vi "Main Tclk.vi"() -> ()   [LabVIEW 2018] (continued)
                      tunnel: [w9192] -> w9169 mode=indexing
                      tunnel: [w9191] -> w9167 mode=indexing
                      tunnel: [w9190] -> w9166 mode=indexing
                      i -> [w9198]
                      n3011 = for {
                        tunnel: w9204 -> [w9220] mode=indexing
                        tunnel: w9203 -> [w9219] mode=indexing
                        tunnel: w9202 -> [w9218]
                        tunnel: w9201 -> [w9217] mode=indexing
                        tunnel: w9200 -> [w9216]
                        tunnel: [w9215] -> w9199 mode=indexing
                        tunnel: w9198 -> [w9214]
                        tunnel: [w9212] -> w9197 mode=indexing
                        tunnel: [w9211] -> w9196 mode=indexing
                        tunnel: [w9210] -> w9195 mode=indexing
                        tunnel: [w9209] -> w9194 mode=indexing
                        tunnel: w9193 -> [w9208]
                        tunnel: [w9207] -> w9192 mode=indexing
                        tunnel: [w9206] -> w9191 mode=indexing
                        tunnel: [w9205] -> w9190 mode=indexing
                        i -> [w9213]
                        n3012 = stacked-sequence {
                          seq-local: [w9223 _ _] -> [_ w9261 _]
                          seq-local: [w9221 _ _] -> [_ w9252 _]
                          tunnel: w9220 -> [w9228 w9253 w9308]
                          tunnel: w9219 -> [w9227 w9266 w9307]
                          tunnel: w9218 -> [w9225 w9249 _]
                          tunnel: w9217 -> [w9222 _ _]
                          tunnel: w9216 -> [w9224 w9250 _]
                          tunnel: [_ w9262 _] -> w9215
                          tunnel: w9214 -> [_ w9260 _]
                          tunnel: w9213 -> [_ w9259 _]
                          tunnel: [w9221 _ _] -> w9212
                          tunnel: [_ w9258 _] -> w9211
                          tunnel: [_ w9257 _] -> w9210
                          tunnel: [_ w9256 _] -> w9209
                          tunnel: w9208 -> [_ w9255 _]
                          tunnel: [_ w9254 _] -> w9207
                          tunnel: [_ w9251 _] -> w9206
                          tunnel: [_ _ w9306] -> w9205
                          frame #0 {
                            n3013 = Subtract(x=w9224, y=w9222) -> (x-y=w9226:u8)
                            n3014 = Less?(x=w9225, y=w9226) -> (x < y?=w9229:bool)
                            n3015 = case shown="True" w9229 {
                              tunnel: w9228 -> [w9231 w9236]
                              tunnel: w9225 -> [_ w9235]
                              tunnel: w9227 -> [_ w9237]
                              tunnel: [w9231 w9234] -> w9223
                              tunnel: w9222 -> [w9230 w9233]
                              tunnel: [w9230 w9232] -> w9221
                              frame False {
                              }
                              frame True {
                                n3016 = Index Array(array=w9236, index=w9235) -> (element=w9239:sgl)
                                n3017 = call "1D Parabolic Max.vi"("Y"=w9237, "Xt"=w9239, "X"=w9236) -> ("Y(Xt) < Ymin"=w9238:bool)  [unwired: 1 in, 7 out]
                                n3018 = case shown="False" w9238 {
                                tunnel: w9235 -> [_ w9245]
                                tunnel: w9236 -> [w9241 w9246]
                                tunnel: w9233 -> [w9240 w9243]
                                tunnel: [w9241 w9244] -> w9234
                                tunnel: [w9240 w9242] -> w9232
                                frame False {
                                }
                                frame True {
                                n3019 = Delete From Array(array=w9246, length=1, index=w9245) -> (array with subset deleted=w9244:sgl[])  [unwired: 1 out]
                                n3020 = Increment(x=w9243) -> (x+1=w9242:u8)
                                }
                                }
                              }
                            }
                          }
                          frame #1 {
                            n3021 = Subtract(x=w9250, y=w9252) -> (x-y=w9265:u8)
                            n3022 = call "1D Parabolic Max.vi"("Y"=w9266, "X"=w9253) -> ("Found max"=w9256:bool, "Ymax"=w9263:dbl, "Xmax"=w9267:dbl, "Finer Best Polynomial Fit"=w9269:dbl[], "Finer X"=w9264:dbl[])  [unwired: 2 in, 3 out]
                            n3023 = Greater Or Equal?(x=w9249, y=w9265) -> (x >= y?=w9268:bool)
                            n3024 = Subtract(x=w9250, y=w9249) -> (x-y=w9248:u8)
                            n3025 = Compound Arithmetic op=OR(w9256, w9268, w9255) -> (w9254:bool)
                            n3026 = case shown="True" w9254 {
                              tunnel: w9267 -> [_ w9287]
                              tunnel: w9266 -> [w9271 w9299]
                              tunnel: w9261 -> [w9279 _]
                              tunnel: w9269 -> [_ w9298]
                              tunnel: w9264 -> [_ w9297]
                              tunnel: w9263 -> [_ w9288]
                              tunnel: w9248 -> [_ w9296]
                              tunnel: w9249 -> [_ w9294]
                              tunnel: [w9279 w9293] -> w9262
                              tunnel: w9260 -> [w9276 w9284]
                              tunnel: w9259 -> [w9277 w9283]
                              tunnel: [w9270 w9288] -> w9258
                              tunnel: [w9274 w9287] -> w9257
                              tunnel: w9253 -> [w9275 w9286]
                              tunnel: [w9278 w9285] -> w9251
                              frame False {
                                n3027 = Build Cluster Array(w9275, w9271) -> (w9280:cluster{"Center":sgl, "A Img Focus Index":sgl}[])
                                n3028 = Sort 1D Array(array=w9280) -> (sorted array=w9281:cluster{"Center":sgl, "A Img Focus Index":sgl}[])
                                n3029 = Bundle(w9281) -> (w9282:T73)  [unwired: 1 in]
                                n3030 = Build Array(w9282) -> (w9278:T74)
                                n3031 = local write "AAX Y tile"(w9276) -> ()
                                n3032 = local write "AAX X tile"(w9277) -> ()
                                n3033 = local write "Auto Aln X"(w9278) -> ()
                                n3034 = Index Array(array=w9275, index=0) -> (element=w9274:sgl)
                                n3035 = Index Array(array=w9271, index=0) -> (element=w9270:sgl)
                              }
                              frame True {
                                n3036 = local read "SEM Scan Parameters"() -> (w9291:T26)
                                n3037 = Initialize Array(w9287, w9296) -> (w9295:dbl[])
                                n3038 = Replace Array Subset(array=w9286, new element=w9295, index=w9294) -> (w9293:sgl[])
                                n3039 = Build Cluster Array(w9286, w9299) -> (w9304:cluster{"Center":sgl, "A Img Focus Index":sgl}[])
                                n3040 = Build Cluster Array(w9297, w9298) -> (w9301:cluster{dbl, dbl}[])
                                n3041 = local write "AAX Y tile"(w9284) -> ()
                                n3042 = local write "AAX X tile"(w9283) -> ()
                                n3043 = Unbundle By Name(w9291) -> ("X aln"=w9292:sgl[][])
                                n3044 = Sort 1D Array(array=w9304) -> (sorted array=w9303:cluster{"Center":sgl, "A Img Focus Index":sgl}[])
                                n3045 = Sort 1D Array(array=w9301) -> (sorted array=w9302:cluster{dbl, dbl}[])
                                n3046 = Replace Array Subset(array=w9292, new element=w9287, index (row)=w9284, index (col)=w9283) -> (w9290:sgl[][])
                                n3047 = Bundle(w9303) -> (w9305:T73)  [unwired: 1 in]
                                n3048 = Bundle(w9302) -> (w9300:cluster{cluster{dbl, dbl}[]})  [unwired: 1 in]
                                n3049 = Bundle By Name(cluster=w9291, "X aln"=w9290) -> (w9289:T26)
                                n3050 = local write "SEM Scan Parameters"(w9289) -> ()
                                n3051 = Build Array(w9305, w9300) -> (w9285:T75)
                                n3052 = local write "Auto Aln X"(w9285) -> ()
                              }
                            }
                          }
                          frame #2 {
                            n3053 = Array Size(array=w9307) -> (size(s)=w9310:i32)
                            n3054 = Greater Or Equal?(x=w9310, y=2) -> (x >= y?=w9311:bool)
                            n3055 = Array Subset(array=w9308, length=w9310) -> (w9309:sgl[])  [unwired: 1 in]
                            n3056 = case shown="True" w9311 {
                              tunnel: w9307 -> [_ w9323]
                              tunnel: w9309 -> [_ w9319]
                              tunnel: [_ w9313] -> w9306
                              frame False {
                              }
                              frame True {
                                n3057 = Array Max & Min(array=w9319) -> (max value=w9321:sgl, min value=w9320:sgl)  [unwired: 2 out]
                                n3058 = Array Max & Min(array=w9323) -> (max value=w9325:sgl, min value=w9326:sgl)  [unwired: 2 out]
                                n3059 = Subtract(x=w9321, y=w9320) -> (x-y=w9322:sgl)
                                n3060 = Subtract(x=w9325, y=w9326) -> (x-y=w9324:sgl)
                                n3061 = expression code="x*0.2"(w9322) -> (w9318:sgl)
                                n3062 = expression code="x*0.2"(w9324) -> (w9327:sgl)
                                n3063 = Add(x=w9321, y=w9318) -> (x+y=w9317:sgl)
                                n3064 = Subtract(x=w9320, y=w9318) -> (x-y=w9316:sgl)
                                n3065 = Add(x=w9325, y=w9327) -> (x+y=w9315:sgl)
                                n3066 = Subtract(x=w9326, y=w9327) -> (x-y=w9314:sgl)
                                n3067 = Bundle(w9317, w9316, w9315, w9314) -> (w9313:cluster{sgl, sgl, sgl, sgl})  [unwired: 1 in]
                                n3068 = property on="Auto Aln X" class="XYGraph (strict)"("XScale.Maximum"=w9317, "XScale.Minimum"=w9316, "YScale.Maximum"=w9315, "YScale.Minimum"=w9314) -> ()  [unwired: 2 in, 2 out]
                              }
                            }
                          }
                        }
                      }
                    }
                    n3069 = And Array Elements(Boolean array=w9169) -> (logical AND=w9168:bool)
                    n3070 = local write "AAX Success tiled"(w9171) -> ()
                    n3071 = local write "AAX Graph scales tiled"(w9166) -> ()
                    n3072 = local write "AlnX array tiled"(w9175) -> ()
                    n3073 = local write "AAX Graph tiled"(w9167) -> ()
                    n3074 = local write "Best Aln X FI tiled"(w9173) -> ()
                    n3075 = local write "Skip Steps tiled"(w9174) -> ()
                    n3076 = local write "Best Aln X (%) tiled"(w9172) -> ()
                    n3077 = case shown="True" w9168 {
                      frame False {
                      }
                      frame True {
                        w9187 = T44."Enabled" ("Disabled")
                        w9189 = sgl[][][] [] ("FI array tiled")
                        n3078 = local read "SEM Scan Parameters"() -> (w9186:T26)
                        n3079 = Unbundle By Name(w9186) -> ("Y tiles"=w9182:u8, "X tiles"=w9183:u8)
                        n3080 = local write "AA Count"(u8 0 ("AA Count")) -> ()
                        n3081 = local write "FI array tiled"(w9189) -> ()
                        n3082 = local write "AlnX array tiled"(w9189) -> ()
                        n3083 = local write "Aln Options"(enum16{"Defaut", "Aln X", "Aln Y"}."Aln Y" ("Aln Options")) -> ()
                        n3084 = property on="Auto Align" class="Bool (strict)"("DisabledEnum"=w9187) -> ()  [unwired: 2 in, 2 out]
                        n3085 = property on="AA Steps" class="DigNum (strict)"("DisabledEnum"=w9187) -> ()  [unwired: 2 in, 2 out]
                        n3086 = Initialize Array(u8 0 ("Skip Steps"), w9182, w9183) -> (w9184:u8[][])
                        n3087 = local write "Skip Steps tiled"(w9184) -> ()
                      }
                    }
                  }
                  frame True {
                  }
                }
              }
              frame #35 {
                n3088 = local read "AlnY array tiled"() -> (w9329:sgl[][][])
                n3089 = local read "FI array tiled"() -> (w9330:sgl[][][])
                n3090 = local read "AA Count"() -> (w9331:u8)
                n3091 = local read "AA Steps"() -> (w9333:u8)
                n3092 = local read "Skip Steps tiled"() -> (w9332:u8[][])
                n3093 = local read "Auto Align"() -> (w9334:bool)
                n3094 = Empty Array?(array=w9329) -> (empty?=w9328:bool)
                n3095 = Not(x=w9334) -> (.not. x?=w9335:bool)
                n3096 = case shown="False" w9328 {
                  tunnel: w9329 -> [w9350 _]
                  tunnel: w9330 -> [w9349 _]
                  tunnel: w9331 -> [w9348 _]
                  tunnel: w9332 -> [w9347 _]
                  tunnel: w9333 -> [w9346 _]
                  tunnel: w9335 -> [w9340 _]
                  frame False {
                    n3097 = for {
                      tunnel: w9350 -> [w9371] mode=indexing
                      tunnel: w9349 -> [w9370] mode=indexing
                      tunnel: w9348 -> [w9369]
                      tunnel: w9347 -> [w9368] mode=indexing
                      tunnel: w9346 -> [w9367]
                      tunnel: [w9366] -> w9345 mode=indexing
                      tunnel: [w9364] -> w9344 mode=indexing
                      tunnel: [w9363] -> w9343 mode=indexing
                      tunnel: [w9362] -> w9342 mode=indexing
                      tunnel: [w9361] -> w9341 mode=indexing
                      tunnel: w9340 -> [w9360]
                      tunnel: [w9359] -> w9339 mode=indexing
                      tunnel: [w9358] -> w9337 mode=indexing
                      tunnel: [w9357] -> w9336 mode=indexing
                      i -> [w9365]
                      n3098 = for {
                        tunnel: w9371 -> [w9387] mode=indexing
                        tunnel: w9370 -> [w9386] mode=indexing
                        tunnel: w9369 -> [w9385]
                        tunnel: w9368 -> [w9384] mode=indexing
                        tunnel: w9367 -> [w9383]
                        tunnel: [w9382] -> w9366 mode=indexing
                        tunnel: w9365 -> [w9381]
                        tunnel: [w9379] -> w9364 mode=indexing
                        tunnel: [w9378] -> w9363 mode=indexing
                        tunnel: [w9377] -> w9362 mode=indexing
                        tunnel: [w9376] -> w9361 mode=indexing
                        tunnel: w9360 -> [w9375]
                        tunnel: [w9374] -> w9359 mode=indexing
                        tunnel: [w9373] -> w9358 mode=indexing
                        tunnel: [w9372] -> w9357 mode=indexing
                        i -> [w9380]
                        n3099 = stacked-sequence {
                          seq-local: [w9390 _ _] -> [_ w9428 _]
                          seq-local: [w9388 _ _] -> [_ w9419 _]
                          tunnel: w9387 -> [w9395 w9420 w9475]
                          tunnel: w9386 -> [w9394 w9433 w9474]
                          tunnel: w9385 -> [w9392 w9416 _]
                          tunnel: w9384 -> [w9389 _ _]
                          tunnel: w9383 -> [w9391 w9417 _]
                          tunnel: [_ w9429 _] -> w9382
                          tunnel: w9381 -> [_ w9427 _]
                          tunnel: w9380 -> [_ w9426 _]
                          tunnel: [w9388 _ _] -> w9379
                          tunnel: [_ w9425 _] -> w9378
                          tunnel: [_ w9424 _] -> w9377
                          tunnel: [_ w9423 _] -> w9376
                          tunnel: w9375 -> [_ w9422 _]
                          tunnel: [_ w9421 _] -> w9374
                          tunnel: [_ w9418 _] -> w9373
                          tunnel: [_ _ w9473] -> w9372
                          frame #0 {
                            n3100 = Subtract(x=w9391, y=w9389) -> (x-y=w9393:u8)
                            n3101 = Less?(x=w9392, y=w9393) -> (x < y?=w9396:bool)
                            n3102 = case shown="True" w9396 {
                              tunnel: w9395 -> [w9398 w9403]
                              tunnel: w9392 -> [_ w9402]
                              tunnel: w9394 -> [_ w9404]
                              tunnel: [w9398 w9401] -> w9390
                              tunnel: w9389 -> [w9397 w9400]
                              tunnel: [w9397 w9399] -> w9388
                              frame False {
                              }
                              frame True {
                                n3103 = Index Array(array=w9403, index=w9402) -> (element=w9406:sgl)
                                n3104 = call "1D Parabolic Max.vi"("Y"=w9404, "Xt"=w9406, "X"=w9403) -> ("Y(Xt) < Ymin"=w9405:bool)  [unwired: 1 in, 7 out]
                                n3105 = case shown="True" w9405 {
                                tunnel: w9402 -> [_ w9412]
                                tunnel: w9403 -> [w9408 w9413]
                                tunnel: w9400 -> [w9407 w9410]
                                tunnel: [w9408 w9411] -> w9401
                                tunnel: [w9407 w9409] -> w9399
                                frame False {
                                }
                                frame True {
                                n3106 = Delete From Array(array=w9413, length=1, index=w9412) -> (array with subset deleted=w9411:sgl[])  [unwired: 1 out]
                                n3107 = Increment(x=w9410) -> (x+1=w9409:u8)
                                }
                                }
                              }
                            }
                          }
                          frame #1 {
                            n3108 = Subtract(x=w9417, y=w9419) -> (x-y=w9432:u8)
                            n3109 = call "1D Parabolic Max.vi"("Y"=w9433, "X"=w9420) -> ("Found max"=w9423:bool, "Ymax"=w9430:dbl, "Xmax"=w9434:dbl, "Finer Best Polynomial Fit"=w9436:dbl[], "Finer X"=w9431:dbl[])  [unwired: 2 in, 3 out]
                            n3110 = Greater Or Equal?(x=w9416, y=w9432) -> (x >= y?=w9435:bool)
                            n3111 = Subtract(x=w9417, y=w9416) -> (x-y=w9415:u8)
                            n3112 = Compound Arithmetic op=OR(w9423, w9435, w9422) -> (w9421:bool)
                            n3113 = case shown="True" w9421 {
                              tunnel: w9434 -> [_ w9454]
                              tunnel: w9433 -> [w9438 w9466]
                              tunnel: w9428 -> [w9446 _]
                              tunnel: w9436 -> [_ w9465]
                              tunnel: w9431 -> [_ w9464]
                              tunnel: w9430 -> [_ w9455]
                              tunnel: w9415 -> [_ w9463]
                              tunnel: w9416 -> [_ w9461]
                              tunnel: [w9446 w9460] -> w9429
                              tunnel: w9427 -> [w9443 w9451]
                              tunnel: w9426 -> [w9444 w9450]
                              tunnel: [w9437 w9455] -> w9425
                              tunnel: [w9440 w9454] -> w9424
                              tunnel: w9420 -> [w9441 w9453]
                              tunnel: [w9445 w9452] -> w9418
                              frame False {
                                n3114 = Build Cluster Array(w9441, w9438) -> (w9447:cluster{"Center":sgl, "A Img Focus Index":sgl}[])
                                n3115 = Sort 1D Array(array=w9447) -> (sorted array=w9448:cluster{"Center":sgl, "A Img Focus Index":sgl}[])
                                n3116 = Bundle(w9448) -> (w9449:T73)  [unwired: 1 in]
                                n3117 = Build Array(w9449) -> (w9445:T74)
                                n3118 = local write "AAY Y tile"(w9443) -> ()
                                n3119 = local write "AAY X tile"(w9444) -> ()
                                n3120 = local write "Auto Aln Y"(w9445) -> ()
                                n3121 = Index Array(array=w9441, index=0) -> (element=w9440:sgl)
                                n3122 = Index Array(array=w9438, index=0) -> (element=w9437:sgl)
                              }
                              frame True {
                                n3123 = local read "SEM Scan Parameters"() -> (w9458:T26)
                                n3124 = Initialize Array(w9454, w9463) -> (w9462:dbl[])
                                n3125 = Replace Array Subset(array=w9453, new element=w9462, index=w9461) -> (w9460:sgl[])
                                n3126 = Build Cluster Array(w9453, w9466) -> (w9471:cluster{"Center":sgl, "A Img Focus Index":sgl}[])
                                n3127 = Build Cluster Array(w9464, w9465) -> (w9468:cluster{dbl, dbl}[])
                                n3128 = local write "AAY Y tile"(w9451) -> ()
                                n3129 = local write "AAY X tile"(w9450) -> ()
                                n3130 = Unbundle By Name(w9458) -> ("Y aln"=w9459:sgl[][])
                                n3131 = Sort 1D Array(array=w9471) -> (sorted array=w9470:cluster{"Center":sgl, "A Img Focus Index":sgl}[])
                                n3132 = Sort 1D Array(array=w9468) -> (sorted array=w9469:cluster{dbl, dbl}[])
                                n3133 = Replace Array Subset(array=w9459, new element=w9454, index (row)=w9451, index (col)=w9450) -> (w9457:sgl[][])
                                n3134 = Bundle(w9470) -> (w9472:T73)  [unwired: 1 in]
                                n3135 = Bundle(w9469) -> (w9467:cluster{cluster{dbl, dbl}[]})  [unwired: 1 in]
                                n3136 = Bundle By Name(cluster=w9458, "Y aln"=w9457) -> (w9456:T26)
                                n3137 = local write "SEM Scan Parameters"(w9456) -> ()
                                n3138 = Build Array(w9472, w9467) -> (w9452:T75)
                                n3139 = local write "Auto Aln Y"(w9452) -> ()
                              }
                            }
                          }
                          frame #2 {
                            n3140 = Array Size(array=w9474) -> (size(s)=w9477:i32)
                            n3141 = Greater Or Equal?(x=w9477, y=2) -> (x >= y?=w9478:bool)
                            n3142 = Array Subset(array=w9475, length=w9477) -> (w9476:sgl[])  [unwired: 1 in]
                            n3143 = case shown="True" w9478 {
                              tunnel: w9474 -> [_ w9490]
                              tunnel: w9476 -> [_ w9486]
                              tunnel: [_ w9480] -> w9473
                              frame False {
                              }
                              frame True {
                                n3144 = Array Max & Min(array=w9486) -> (max value=w9488:sgl, min value=w9487:sgl)  [unwired: 2 out]
                                n3145 = Array Max & Min(array=w9490) -> (max value=w9492:sgl, min value=w9493:sgl)  [unwired: 2 out]
                                n3146 = Subtract(x=w9488, y=w9487) -> (x-y=w9489:sgl)
                                n3147 = Subtract(x=w9492, y=w9493) -> (x-y=w9491:sgl)
                                n3148 = expression code="x*0.2"(w9489) -> (w9485:sgl)
                                n3149 = expression code="x*0.2"(w9491) -> (w9494:sgl)
                                n3150 = Add(x=w9488, y=w9485) -> (x+y=w9484:sgl)
                                n3151 = Subtract(x=w9487, y=w9485) -> (x-y=w9483:sgl)
                                n3152 = Add(x=w9492, y=w9494) -> (x+y=w9482:sgl)
                                n3153 = Subtract(x=w9493, y=w9494) -> (x-y=w9481:sgl)
                                n3154 = Bundle(w9484, w9483, w9482, w9481) -> (w9480:cluster{sgl, sgl, sgl, sgl})  [unwired: 1 in]
                                n3155 = property on="Auto Aln Y" class="XYGraph (strict)"("XScale.Maximum"=w9484, "XScale.Minimum"=w9483, "YScale.Maximum"=w9482, "YScale.Minimum"=w9481) -> ()  [unwired: 2 in, 2 out]
                              }
                            }
                          }
                        }
                      }
                    }
                    n3156 = And Array Elements(Boolean array=w9339) -> (logical AND=w9338:bool)
                    n3157 = local write "AAY Success tiled"(w9341) -> ()
                    n3158 = local write "AAY Graph scales tiled"(w9336) -> ()
                    n3159 = local write "AlnY array tiled"(w9345) -> ()
                    n3160 = local write "AAY Graph tiled"(w9337) -> ()
                    n3161 = local write "Best Aln Y FI tiled"(w9343) -> ()
                    n3162 = local write "Skip Steps tiled"(w9344) -> ()
                    n3163 = local write "Best Aln Y (%) tiled"(w9342) -> ()
                    n3164 = case shown="True" w9338 {
                      frame False {
                      }
                      frame True {
                        w9353 = T44."Enabled" ("Disabled")
                        w9355 = sgl[][][] [] ("FI array tiled")
                        n3165 = local write "Auto Align"(FALSE ("Auto Stig")) -> ()
                        n3166 = local write "AA Count"(u8 0 ("AA Count")) -> ()
                        n3167 = local write "Skip Steps tiled"(u8[][] [] ("AS Count tiled")) -> ()
                        n3168 = local write "FI array tiled"(w9355) -> ()
                        n3169 = local write "AlnX array tiled"(w9355) -> ()
                        n3170 = local write "Aln Options"(enum16{"Defaut", "Aln X", "Aln Y"}."Defaut" ("Aln Options")) -> ()
                        n3171 = property on="Auto Focus" class="Bool (strict)"("DisabledEnum"=w9353) -> ()  [unwired: 2 in, 2 out]
                        n3172 = property on="Auto Stig" class="Bool (strict)"("DisabledEnum"=w9353) -> ()  [unwired: 2 in, 2 out]
                        n3173 = property on="Auto Align" class="Bool (strict)"("DisabledEnum"=w9353) -> ()  [unwired: 2 in, 2 out]
                        n3174 = property on="AA Steps" class="DigNum (strict)"("DisabledEnum"=w9353) -> ()  [unwired: 2 in, 2 out]
                      }
                    }
                  }
                  frame True {
                  }
                }
              }
              frame #36 {
                n3175 = local read "Low Mag SEM"() -> (w9495:T30)
                n3176 = local read "Mid Mag SEM"() -> (w9496:T29)
                n3177 = Unbundle By Name(w9495) -> ("Low mag scan"=w9497:bool)
                n3178 = Unbundle By Name(w9496) -> ("Mid mag scan"=w9498:bool)
                n3179 = case shown="True" w9497 {
                  tunnel: w9495 -> [_ w9521]
                  frame False {
                  }
                  frame True {
                    w9517 = sgl[] [0.0] ("dX (um)")
                    w9518 = u8 1 ("X tiles")
                    w9522 = 0.0 ("X center")
                    n3180 = Unbundle By Name(w9521) -> ("Low mag scan FOV (micron)"=w9519:dbl, "Low mag scan rate (Hz)"=w9531:u32)
                    n3181 = local read "SEM Scan Parameters"() -> (w9524:T26)
                    n3182 = Unbundle By Name(w9524) -> ("Scan rate (Hz)"=w9526:u32, "Oversampling"=w9525:u32)
                    n3183 = expression code="x*1000"(w9519) -> (w9532:dbl)
                    n3184 = Multiply(x=w9526, y=w9525) -> (x*y=w9527:u32)
                    n3185 = Divide(x=w9527, y=w9531) -> (x/y=w9528:dbl)
                    n3186 = Divide(x=w9532, y=u32 512 ("X resolution")) -> (x/y=w9530:dbl)
                    n3187 = Bundle By Name(cluster=w9524, "X size (um)"=w9519, "Y size (um)"=w9519, "X center (um)"=w9522, "Y center (um)"=w9522, "X size (V)"=20.0, "Scan rate (Hz)"=w9531, "Oversampling"=w9528, "X tiles"=w9518, "Y tiles"=w9518, "Frames"=w9518, "dX (um)"=w9517, "dY (um)"=w9517, "Pixel size (nm)"=w9530) -> (w9520:T26)
                    n3188 = local write "SEM Low Mag Scan Parameters"(w9520) -> ()
                  }
                }
                n3189 = case shown="True" w9498 {
                  tunnel: w9496 -> [_ w9505]
                  frame False {
                  }
                  frame True {
                    w9499 = sgl[] [0.0] ("dX (um)")
                    w9500 = u8 1 ("X tiles")
                    n3190 = Unbundle By Name(w9505) -> ("X size (um)"=w9511:sgl, "Y size (um)"=w9510:sgl, "X center (um)"=w9509:dbl, "Y center (um)"=w9508:dbl, "Mid mag scan rate (Hz)"=w9507:u32, "Pixel size (nm)"=w9506:sgl)
                    n3191 = local read "SEM Mid Mag Scan Parameters"() -> (w9503:T5)
                    n3192 = local read "SEM Scan Parameters"() -> (w9512:T26)
                    n3193 = Unbundle By Name(w9512) -> ("Scan rate (Hz)"=w9514:u32, "Oversampling"=w9513:u32)
                    n3194 = Unbundle By Name(w9503) -> ("X size (V)"=w9502:dbl)
                    n3195 = Multiply(x=w9514, y=w9513) -> (x*y=w9515:u32)
                    n3196 = Divide(x=w9515, y=w9507) -> (x/y=w9516:dbl)
                    n3197 = Bundle By Name(cluster=w9512, "X size (um)"=w9511, "Y size (um)"=w9510, "X center (um)"=w9509, "Y center (um)"=w9508, "Oversampling auto"=TRUE ("X size auto"), "Scan rate (Hz)"=w9507, "Oversampling"=w9516, "Pixel size (nm)"=w9506, "X size (V)"=w9502, "X tiles"=w9500, "Y tiles"=w9500, "Frames"=w9500, "dX (um)"=w9499, "dY (um)"=w9499) -> (w9501:T26)
                    n3198 = local write "SEM Mid Mag Scan Parameters"(w9501) -> ()
                  }
                }
              }
              frame #37 {
                n3199 = local read "Mid Mag SEM"() -> (w9547:T29)
                n3200 = local read "FIB slice #"() -> (w9541:u32)
                n3201 = Unbundle By Name(w9547) -> ("Mid mag scan"=w9548:bool, "Prior to main scan"=w9549:bool, "Mid mag interval"=w9535:u32)
                n3202 = Equal?(x=u32 1 ("y"), y=w9535) -> (x = y?=w9539:bool)
                n3203 = case shown="False" w9539 {
                  tunnel: [w9553 w9556] -> w9537
                  tunnel: [w9552 w9556] -> w9538
                  tunnel: [w9550 w9556] -> w9536
                  frame False {
                    n3204 = local read "Auto Focus"() -> (w9555:bool)
                    n3205 = local read "Auto Stig"() -> (w9554:bool)
                    n3206 = local read "Auto Align"() -> (w9551:bool)
                    n3207 = Not(x=w9555) -> (.not. x?=w9552:bool)
                    n3208 = Not(x=w9554) -> (.not. x?=w9553:bool)
                    n3209 = Not(x=w9551) -> (.not. x?=w9550:bool)
                  }
                  frame True {
                    w9556 = TRUE
                  }
                }
                n3210 = Subtract(x=w9541, y=u32 2) -> (x-y=w9533:u32)
                n3211 = Quotient & Remainder(x=w9533, y=w9535) -> (x-y*floor(x/y)=w9545:u32)  [unwired: 1 out]
                n3212 = local read "FIB"() -> (w9542:bool)
                n3213 = Not(x=w9549) -> (.not. x?=w9544:bool)
                n3214 = Equal To 0?(x=w9545) -> (x = 0?=w9546:bool)
                n3215 = Compound Arithmetic op=AND(w9542, w9538, w9537, w9536, w9548, w9544, w9546) -> (w9543:bool)
                n3216 = case shown="True" w9543 {
                  frame False {
                    n3217 = local write "Mid Mag SEM on"(FALSE ("Mid Mag SEM on")) -> ()
                    n3218 = local write "MM overhead"(u32 0 ("MM overhead")) -> ()
                  }
                  frame True {
                    w9570 = FALSE ("GetInfo")
                    n3219 = local read "Tiled scan inputs"() -> (w9569:T6)
                    n3220 = local read "SEM Mid Mag Scan Parameters"() -> (w9568:T5)
                    n3221 = local read "File Information"() -> (w9567:T31)
                    n3222 = local write "Mid Mag SEM on"(TRUE ("Mid Mag SEM on")) -> ()
                    n3223 = Unbundle By Name(w9567) -> ("File path"=w9565:path)
                    n3224 = local write "Status message"("SEM Mid Mag Scan" ("Status message")) -> ()
                    n3225 = local read "MM SEM scan time"() -> (w9562:dbl)
                    n3226 = Build Path(base path=w9565, name or relative path="Mid Mag Scans\\") -> (appended path=w9564:path)
                    n3227 = Bundle By Name(cluster=w9569, "SEM Options.GetInfo"=w9570, "SEM Options.PNG only"=w9570, "SEM Options.Upload"=w9570, "SEM Scan Parameters"=w9568, "File Information.File path"=w9564) -> (w9560:T6)
                    n3228 = local read "WatchDog Mode"() -> (w9561:u16)
                    n3229 = expression code="x+10"(w9562) -> (w9563:dbl)
                    n3230 = local read "Api"() -> (w9559:refnum<k7>)
                    n3231 = local write "MM overhead"(w9563) -> ()
                    n3232 = call "2D scan tiled.vi"("WatchDog Mode"=w9561, "Tiled scan inputs"=w9560, "ActiveX Container"=w9559) -> ()  [unwired: 3 in, 6 out]
                  }
                }
              }
              frame #38 {
                n3233 = local read "Low Mag SEM"() -> (w9578:T30)
                n3234 = local read "FIB slice #"() -> (w9573:u32)
                n3235 = Unbundle By Name(w9578) -> ("Low mag scan"=w9577:bool, "Prior to main scan"=w9576:bool, "Low mag interval"=w9574:u32)
                n3236 = Quotient & Remainder(x=w9573, y=w9574) -> (x-y*floor(x/y)=w9580:u32)  [unwired: 1 out]
                n3237 = local read "FIB"() -> (w9575:bool)
                n3238 = Not(x=w9576) -> (.not. x?=w9581:bool)
                n3239 = Equal To 0?(x=w9580) -> (x = 0?=w9579:bool)
                n3240 = Compound Arithmetic op=AND(w9575, w9577, w9581, w9579) -> (w9582:bool)
                n3241 = case shown="True" w9582 {
                  frame False {
                    n3242 = local write "Low Mag SEM on"(FALSE ("Mid Mag SEM on")) -> ()
                    n3243 = local write "LM overhead"(u32 0 ("LM overhead")) -> ()
                  }
                  frame True {
                    w9592 = FALSE ("GetInfo")
                    n3244 = local read "LM SEM scan time"() -> (w9588:dbl)
                    n3245 = local read "Tiled scan inputs"() -> (w9591:T6)
                    n3246 = local read "SEM Low Mag Scan Parameters"() -> (w9594:T5)
                    n3247 = local read "File Information"() -> (w9595:T31)
                    n3248 = local write "Low Mag SEM on"(TRUE ("Mid Mag SEM on")) -> ()
                    n3249 = Unbundle By Name(w9595) -> ("File path"=w9597:path)
                    n3250 = local write "Status message"("SEM Low Mag Scan" ("Status message")) -> ()
                    n3251 = expression code="x+10"(w9588) -> (w9589:dbl)
                    n3252 = local write "LM overhead"(w9589) -> ()
                    n3253 = Build Path(base path=w9597, name or relative path="Low Mag Scans\\") -> (appended path=w9598:path)
                    n3254 = Bundle By Name(cluster=w9591, "SEM Options.GetInfo"=w9592, "SEM Options.PNG only"=TRUE ("PNG only"), "SEM Options.Upload"=w9592, "SEM Scan Parameters"=w9594, "File Information.File path"=w9598) -> (w9586:T6)
                    n3255 = local read "WatchDog Mode"() -> (w9587:u16)
                    n3256 = local read "Api"() -> (w9585:refnum<k7>)
                    n3257 = call "2D scan tiled.vi"("WatchDog Mode"=w9587, "Tiled scan inputs"=w9586, "ActiveX Container"=w9585) -> ()  [unwired: 3 in, 6 out]
                  }
                }
              }
              frame #39 {
                n3258 = local read "Low Mag SEM"() -> (w9616:T30)
                n3259 = local read "FIB slice #"() -> (w9613:u32)
                n3260 = local read "FIB HW Config"() -> (w9619:T23)
                n3261 = Unbundle By Name(w9616) -> ("Low mag scan"=w9615:bool, "Low mag interval"=w9614:u32)
                n3262 = Unbundle By Name(w9619) -> ("Beam blank"=w9620:tag)
                n3263 = local read "Api"() -> (w9605:refnum<k7>)
                n3264 = Quotient & Remainder(x=w9613, y=w9614) -> (x-y*floor(x/y)=w9618:u32)  [unwired: 1 out]
                n3265 = call "FIB beam blank.vi"("ActiveX Container"=w9605, "Beam blanked"=TRUE, "lines"=w9620) -> ()  [unwired: 2 in, 1 out]
                n3266 = Equal To 0?(x=w9618) -> (x = 0?=w9617:bool)
                n3267 = Compound Arithmetic op=AND(w9615, w9617) -> (w9612:bool)
                n3268 = local read "Last FIB recipe"() -> (w9608:path)
                n3269 = case shown="True" w9612 {
                  frame False {
                  }
                  frame True {
                    n3270 = local read "FIB Image"() -> (w9673:i16[][])
                    n3271 = Array Size(array=w9673) -> (size(s)=w9674:i32[])
                    n3272 = local read "Pre Image"() -> (w9680:i16[][])
                    n3273 = Array Size(array=w9680) -> (size(s)=w9679:i32[])
                    n3274 = Add Array Elements(numeric array=w9674) -> (sum=w9675:i32)
                    n3275 = Add Array Elements(numeric array=w9679) -> (sum=w9678:i32)
                    n3276 = Not Equal To 0?(x=w9675) -> (x != 0?=w9676:bool)
                    n3277 = Not Equal To 0?(x=w9678) -> (x != 0?=w9677:bool)
                    n3278 = case shown="True" w9676 {
                      tunnel: w9673 -> [_ w9700]
                      frame False {
                      }
                      frame True {
                        n3279 = local read "Last FIB image"() -> (w9703:path)
                        n3280 = call "16bit Image Normalization.vi"("Transpose"=FALSE, "Input image"=w9700) -> ("Normalized image"=w9699:u8[][])  [unwired: 5 in, 4 out]
                        n3281 = call <vilib>:"Flatten Pixmap.vi"("colors"=u32[] [16777222, 65793, 131586, 197379, 263172, 328965, 394758, 460551, 526344, 592137, 657930, 723723, 789516, 855309, 921102, 986895, 1052688, 1118481, 1184274, 1250067, 1315860, 1381653, 1447446, 1513239, 1579032, 1644825, 1710618, 1776411, 1842204, 1907997, 1973790, 2039583, 2105376, 2171169, 2236962, 2302755, 2368548, 2434341, 2500134, 2565927, 2631720, 2697513, 2763306, 2829099, 2894892, 2960685, 3026478, 3092271, 3158064, 3223857, 3289650, 3355443, 3421236, 3487029, 3552822, 3618615, 3684408, 3750201, 3815994, 3881787, 3947580, 4013373, 4079166, 4144959, 4210752, 4276545, 4342338, 4408131, 4473924, 4539717, 4605510, 4671303, 4737096, 4802889, 4868682, 4934475, 5000268, 5066061, 5131854, 5197647, 5263440, 5329233, 5395026, 5460819, 5526612, 5592405, 5658198, 5723991, 5789784, 5855577, 5921370, 5987163, 6052956, 6118749, 6184542, 6250335, 6316128, 6381921, 6447714, 6513507, 6579300, 6645093, 6710886, 6776679, 6842472, 6908265, 6974058, 7039851, 7105644, 7171437, 7237230, 7303023, 7368816, 7434609, 7500402, 7566195, 7631988, 7697781, 7763574, 7829367, 7895160, 7960953, 8026746, 8092539, 8158332, 8224125, 8289918, 8355711, 8421504, 8487297, 8553090, 8618883, 8684676, 8750469, 8816262, 8882055, 8947848, 9013641, 9079434, 9145227, 9211020, 9276813, 9342606, 9408399, 9474192, 9539985, 9605778, 9671571, 9737364, 9803157, 9868950, 9934743, 10000536, 10066329, 10132122, 10197915, 10263708, 10329501, 10395294, 10461087, 10526880, 10592673, 10658466, 10724259, 10790052, 10855845, 10921638, 10987431, 11053224, 11119017, 11184810, 11250603, 11316396, 11382189, 11447982, 11513775, 11579568, 11645361, 11711154, 11776947, 11842740, 11908533, 11974326, 12040119, 12105912, 12171705, 12237498, 12303291, 12369084, 12434877, 12500670, 12566463, 12632256, 12698049, 12763842, 12829635, 12895428, 12961221, 13027014, 13092807, 13158600, 13224393, 13290186, 13355979, 13421772, 13487565, 13553358, 13619151, 13684944, 13750737, 13816530, 13882323, 13948116, 14013909, 14079702, 14145495, 14211288, 14277081, 14342874, 14408667, 14474460, 14540253, 14606046, 14671839, 14737632, 14803425, 14869218, 14935011, 15000804, 15066597, 15132390, 15198183, 15263976, 15329769, 15395562, 15461355, 15527148, 15592941, 15658734, 15724527, 15790320, 15856113, 15921906, 15987699, 16053492, 16119285, 16185078, 16250871, 16316664, 16382457, 16448250, 16514043, 16579836, 16645629, 16711422, 16448250] ("256 gray scale"), "8-bit pixmap"=w9699) -> ("image data"=w9702:T52)  [unwired: 4 in, 5 out]
                        n3282 = call <vilib>:"Write PNG File.vi"("image data"=w9702, "path to PNG file"=w9703) -> ()  [unwired: 1 in, 9 out]
                      }
                    }
                    n3283 = case shown="True" w9677 {
                      tunnel: w9680 -> [_ w9694]
                      frame False {
                      }
                      frame True {
                        n3284 = local read "Last FIB zoom pre image"() -> (w9697:path)
                        n3285 = call "16bit Image Normalization.vi"("Transpose"=FALSE, "Input image"=w9694) -> ("Normalized image"=w9693:u8[][])  [unwired: 5 in, 4 out]
                        n3286 = call <vilib>:"Flatten Pixmap.vi"("colors"=u32[] [16777222, 65793, 131586, 197379, 263172, 328965, 394758, 460551, 526344, 592137, 657930, 723723, 789516, 855309, 921102, 986895, 1052688, 1118481, 1184274, 1250067, 1315860, 1381653, 1447446, 1513239, 1579032, 1644825, 1710618, 1776411, 1842204, 1907997, 1973790, 2039583, 2105376, 2171169, 2236962, 2302755, 2368548, 2434341, 2500134, 2565927, 2631720, 2697513, 2763306, 2829099, 2894892, 2960685, 3026478, 3092271, 3158064, 3223857, 3289650, 3355443, 3421236, 3487029, 3552822, 3618615, 3684408, 3750201, 3815994, 3881787, 3947580, 4013373, 4079166, 4144959, 4210752, 4276545, 4342338, 4408131, 4473924, 4539717, 4605510, 4671303, 4737096, 4802889, 4868682, 4934475, 5000268, 5066061, 5131854, 5197647, 5263440, 5329233, 5395026, 5460819, 5526612, 5592405, 5658198, 5723991, 5789784, 5855577, 5921370, 5987163, 6052956, 6118749, 6184542, 6250335, 6316128, 6381921, 6447714, 6513507, 6579300, 6645093, 6710886, 6776679, 6842472, 6908265, 6974058, 7039851, 7105644, 7171437, 7237230, 7303023, 7368816, 7434609, 7500402, 7566195, 7631988, 7697781, 7763574, 7829367, 7895160, 7960953, 8026746, 8092539, 8158332, 8224125, 8289918, 8355711, 8421504, 8487297, 8553090, 8618883, 8684676, 8750469, 8816262, 8882055, 8947848, 9013641, 9079434, 9145227, 9211020, 9276813, 9342606, 9408399, 9474192, 9539985, 9605778, 9671571, 9737364, 9803157, 9868950, 9934743, 10000536, 10066329, 10132122, 10197915, 10263708, 10329501, 10395294, 10461087, 10526880, 10592673, 10658466, 10724259, 10790052, 10855845, 10921638, 10987431, 11053224, 11119017, 11184810, 11250603, 11316396, 11382189, 11447982, 11513775, 11579568, 11645361, 11711154, 11776947, 11842740, 11908533, 11974326, 12040119, 12105912, 12171705, 12237498, 12303291, 12369084, 12434877, 12500670, 12566463, 12632256, 12698049, 12763842, 12829635, 12895428, 12961221, 13027014, 13092807, 13158600, 13224393, 13290186, 13355979, 13421772, 13487565, 13553358, 13619151, 13684944, 13750737, 13816530, 13882323, 13948116, 14013909, 14079702, 14145495, 14211288, 14277081, 14342874, 14408667, 14474460, 14540253, 14606046, 14671839, 14737632, 14803425, 14869218, 14935011, 15000804, 15066597, 15132390, 15198183, 15263976, 15329769, 15395562, 15461355, 15527148, 15592941, 15658734, 15724527, 15790320, 15856113, 15921906, 15987699, 16053492, 16119285, 16185078, 16250871, 16316664, 16382457, 16448250, 16514043, 16579836, 16645629, 16711422, 16448250] ("256 gray scale"), "8-bit pixmap"=w9693) -> ("image data"=w9696:T52)  [unwired: 4 in, 5 out]
                        n3287 = call <vilib>:"Write PNG File.vi"("image data"=w9696, "path to PNG file"=w9697) -> ()  [unwired: 1 in, 9 out]
                      }
                    }
                    n3288 = local read "Detector A Low Mag"() -> (w9671:i16[][])
                    n3289 = local read "Detector B Low Mag"() -> (w9672:i16[][])
                    n3290 = Array Size(array=w9671) -> (size(s)=w9670:i32[])
                    n3291 = Array Size(array=w9672) -> (size(s)=w9665:i32[])
                    n3292 = Add Array Elements(numeric array=w9670) -> (sum=w9669:i32)
                    n3293 = Add Array Elements(numeric array=w9665) -> (sum=w9666:i32)
                    n3294 = Not Equal To 0?(x=w9669) -> (x != 0?=w9668:bool)
                    n3295 = Not Equal To 0?(x=w9666) -> (x != 0?=w9667:bool)
                    n3296 = case shown="True" w9668 {
                      tunnel: w9671 -> [_ w9688]
                      frame False {
                      }
                      frame True {
                        n3297 = local read "Last Det A Low Mag"() -> (w9691:path)
                        n3298 = call "16bit Image Normalization.vi"("Transpose"=FALSE, "Input image"=w9688) -> ("Normalized image"=w9687:u8[][])  [unwired: 5 in, 4 out]
                        n3299 = call <vilib>:"Flatten Pixmap.vi"("colors"=u32[] [16777222, 65793, 131586, 197379, 263172, 328965, 394758, 460551, 526344, 592137, 657930, 723723, 789516, 855309, 921102, 986895, 1052688, 1118481, 1184274, 1250067, 1315860, 1381653, 1447446, 1513239, 1579032, 1644825, 1710618, 1776411, 1842204, 1907997, 1973790, 2039583, 2105376, 2171169, 2236962, 2302755, 2368548, 2434341, 2500134, 2565927, 2631720, 2697513, 2763306, 2829099, 2894892, 2960685, 3026478, 3092271, 3158064, 3223857, 3289650, 3355443, 3421236, 3487029, 3552822, 3618615, 3684408, 3750201, 3815994, 3881787, 3947580, 4013373, 4079166, 4144959, 4210752, 4276545, 4342338, 4408131, 4473924, 4539717, 4605510, 4671303, 4737096, 4802889, 4868682, 4934475, 5000268, 5066061, 5131854, 5197647, 5263440, 5329233, 5395026, 5460819, 5526612, 5592405, 5658198, 5723991, 5789784, 5855577, 5921370, 5987163, 6052956, 6118749, 6184542, 6250335, 6316128, 6381921, 6447714, 6513507, 6579300, 6645093, 6710886, 6776679, 6842472, 6908265, 6974058, 7039851, 7105644, 7171437, 7237230, 7303023, 7368816, 7434609, 7500402, 7566195, 7631988, 7697781, 7763574, 7829367, 7895160, 7960953, 8026746, 8092539, 8158332, 8224125, 8289918, 8355711, 8421504, 8487297, 8553090, 8618883, 8684676, 8750469, 8816262, 8882055, 8947848, 9013641, 9079434, 9145227, 9211020, 9276813, 9342606, 9408399, 9474192, 9539985, 9605778, 9671571, 9737364, 9803157, 9868950, 9934743, 10000536, 10066329, 10132122, 10197915, 10263708, 10329501, 10395294, 10461087, 10526880, 10592673, 10658466, 10724259, 10790052, 10855845, 10921638, 10987431, 11053224, 11119017, 11184810, 11250603, 11316396, 11382189, 11447982, 11513775, 11579568, 11645361, 11711154, 11776947, 11842740, 11908533, 11974326, 12040119, 12105912, 12171705, 12237498, 12303291, 12369084, 12434877, 12500670, 12566463, 12632256, 12698049, 12763842, 12829635, 12895428, 12961221, 13027014, 13092807, 13158600, 13224393, 13290186, 13355979, 13421772, 13487565, 13553358, 13619151, 13684944, 13750737, 13816530, 13882323, 13948116, 14013909, 14079702, 14145495, 14211288, 14277081, 14342874, 14408667, 14474460, 14540253, 14606046, 14671839, 14737632, 14803425, 14869218, 14935011, 15000804, 15066597, 15132390, 15198183, 15263976, 15329769, 15395562, 15461355, 15527148, 15592941, 15658734, 15724527, 15790320, 15856113, 15921906, 15987699, 16053492, 16119285, 16185078, 16250871, 16316664, 16382457, 16448250, 16514043, 16579836, 16645629, 16711422, 16448250] ("256 gray scale"), "8-bit pixmap"=w9687) -> ("image data"=w9690:T52)  [unwired: 4 in, 5 out]
                        n3300 = call <vilib>:"Write PNG File.vi"("image data"=w9690, "path to PNG file"=w9691) -> ()  [unwired: 1 in, 9 out]
                      }
                    }
                    n3301 = case shown="True" w9667 {
                      tunnel: w9672 -> [_ w9682]
                      frame False {
                      }
                      frame True {
                        n3302 = local read "Last Det B Low Mag"() -> (w9685:path)
                        n3303 = call "16bit Image Normalization.vi"("Transpose"=FALSE, "Input image"=w9682) -> ("Normalized image"=w9681:u8[][])  [unwired: 5 in, 4 out]
